vi "Init.vi"(7 "Prepend Result Name":bool, 8 "error in (no error)":errorcluster, 9 "SA Pin":string, 10 "Measurement Name":string) -> (0 "error out":errorcluster, 3 "NR_ACP out":refnum<class "NR_ACP.lvclass">)   [LabVIEW 2018, in "SeqAuto Evaluations.lvlib" / "NR_ACP.lvclass"]
uses:
  NR_ACP.lvclass
  C:/Seqeunce Automation/Plugins/SeqAuto IEvaluation.lvlibp/SeqAuto IEvaluation.lvclass
  NR_ACP.lvclass/NR_ACP.ctl
  Private Methods/Write SA Pin.vi
  Plugins/SeqAuto IEvaluation.lvlibp/Write Measurement Name.vi
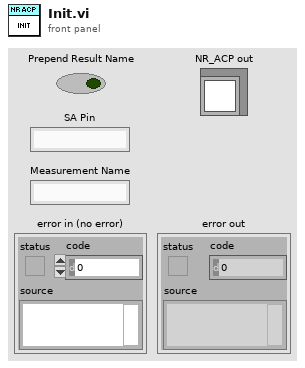
[diagram p1: front panel]
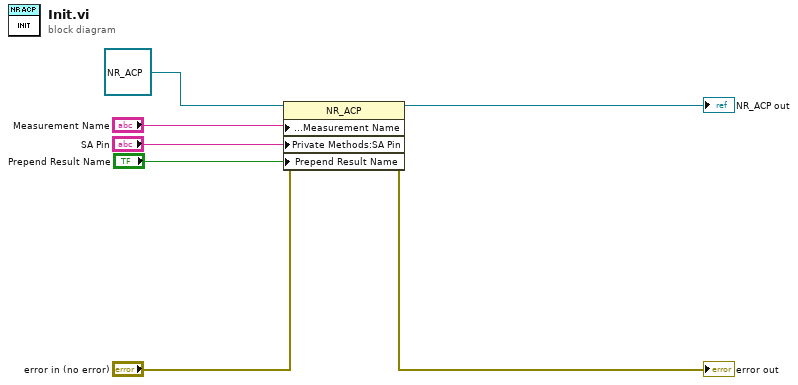
[diagram p0: block diagram]
diagram:
  n1 = property class="NR_ACP"(reference=refnum<class "NR_ACP.lvclass"> refnum ("LTE_ACP in"), error in="error in (no error)", "Protected Methods:Measurement Name"="Measurement Name", "Private Methods:SA Pin"="SA Pin", "Prepend Result Name"="Prepend Result Name") -> (reference out=→"NR_ACP out":refnum<class "NR_ACP.lvclass">, error out=→"error out":errorcluster)
